vi "test u drive access.vi"() -> ()   [LabVIEW 2012]
panel:
  out "error out":errorcluster
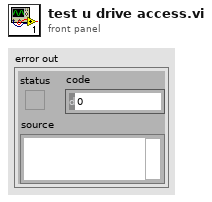
[diagram p1: front panel]
types:
  T1 = enum16{"open", "replace", "create", "open or create", "replace or create", "replace or create with confirmation"}
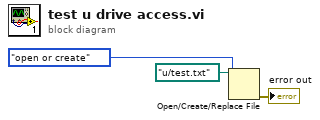
[diagram p0: block diagram]
diagram:
  n1 = Open/Create/Replace File(file path (use dialog)=path "u:/test.txt", operation (0:open)=T1."open or create") -> (error out=→"error out":errorcluster)  [unwired: 4 in, 2 out]
